vi "Read Message.vi"(8 "error in (no error)":errorcluster, 11 "ConfigDTO in":refnum<class "ConfigDTO.lvclass">) -> (0 "error out":errorcluster, 2 "Message":string, 3 "ConfigDTO out":refnum<class "ConfigDTO.lvclass">)   [LabVIEW 2025, in "DataTransitionObjects.lvlib" / "ConfigDTO.lvclass"]
uses:
  ConfigDTO.lvclass
  ConfigDTO.lvclass/ConfigDTO.ctl
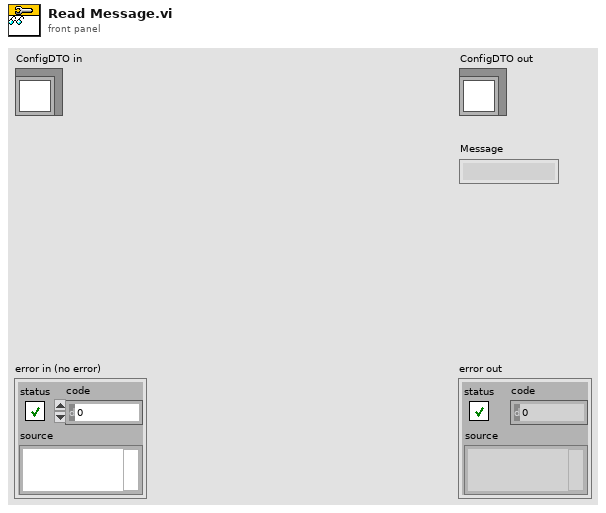
[diagram p1: front panel]
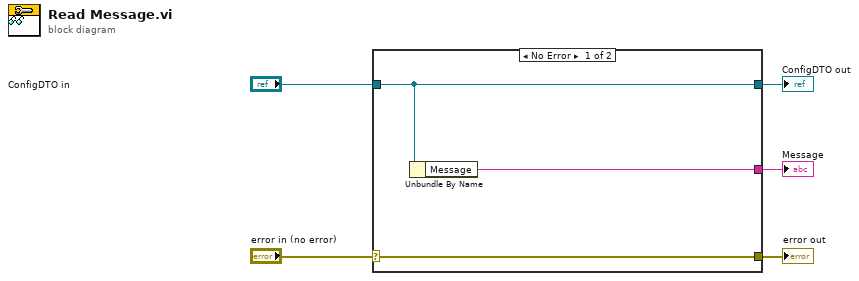
[diagram p0: block diagram]
diagram:
  n1 = case shown="No Error" "error in (no error)" {
    selector: "error in (no error)" -> [w8 w9]
    tunnel: [w8 w9] -> w4
    tunnel: [w7 w10] -> w2
    tunnel: "ConfigDTO in" -> [w7 w10]
    tunnel: [w6 _] -> w1
    frame No Error {
      n2 = Unbundle By Name(w7) -> ("Message"=w6:string)
    }
    frame Error {
    }
  }
  "error out" <- w4
  "ConfigDTO out" <- w2
  "Message" <- w1
